vi "thrower Check for New Command.vi"(8 "Current Command":T6, 10 "Wait time (ms)":dbl, 11 "Finished?":bool) -> (0 "Completion":T4, 1 "Subsystem Name":string, 2 "Current Command":T1, 3 "Initial Trace String":string, 4 "NextCommand":T6)   [LabVIEW 2020]
doc: "This VI is called for each controller loop iteration. It checks for new commands, updates timing data, and upon completion, notifies any waiting commands."
uses:
  thrower Setpoints.ctl
  thrower Operations.ctl
  <vilib>/Rock Robotics/WPI/Framework/Command Status Info.ctl
  <vilib>/Rock Robotics/WPI/Framework/Completion Status.ctl
  <vilib>/Rock Robotics/WPI/Framework/Completion Notifier.ctl
  thrower Published Globals.vi
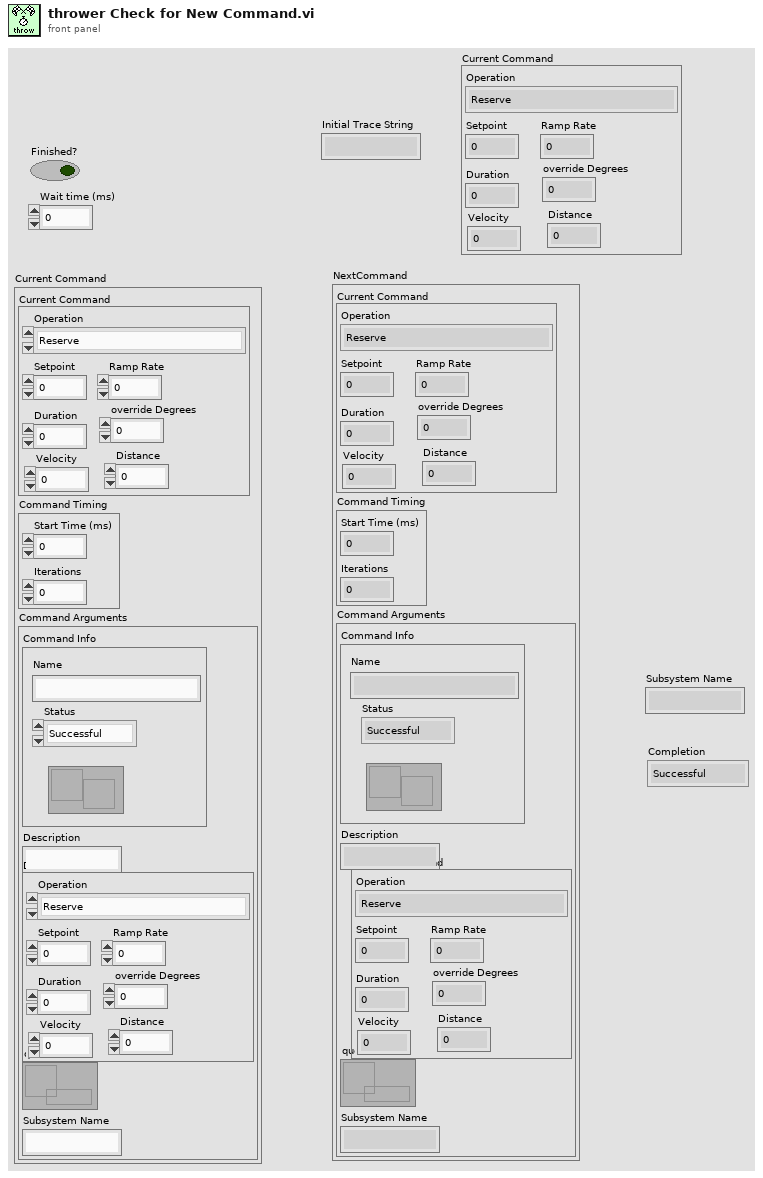
[diagram p1: front panel]
types:
  T1 = typedef "thrower Setpoints.ctl" = cluster{"Operation":T2, "Setpoint":dbl, "Duration":dbl, "Ramp Rate":dbl, "override Degrees":dbl, "Velocity":dbl, "Distance":dbl}
  T2 = typedef "thrower Operations.ctl" = enum16{"Reserve", "Read Current", "Immediate", "feed ball", "rev up thrower", "aim servos", "resetServos", "fire ball"}
  T3 = typedef "Command Status Info.ctl" = cluster{"Name":string, "Status":T4, "notifier out":T5}
  T4 = typedef "Completion Status.ctl" = enum16{"Successful", "Aborted", "Incomplete"}
  T5 = typedef "Completion Notifier.ctl" = refnum<notifier>
  T6 = cluster{"Current Command":T1, "Command Timing":cluster{"Start Time (ms)":u32, "Iterations":i32}, "Command Arguments":cluster{"Command Info":T3, "Description":string, "Default Command":T1, "queue out":refnum<queue>, "Subsystem Name":string}}
  T7 = cluster{"Command Info":T3, "Description":string, "Default Command":T1, "queue out":refnum<queue>, "Subsystem Name":string}
  T8 = cluster{"Default Command":T1, "Command Info":T3, "Description":string}
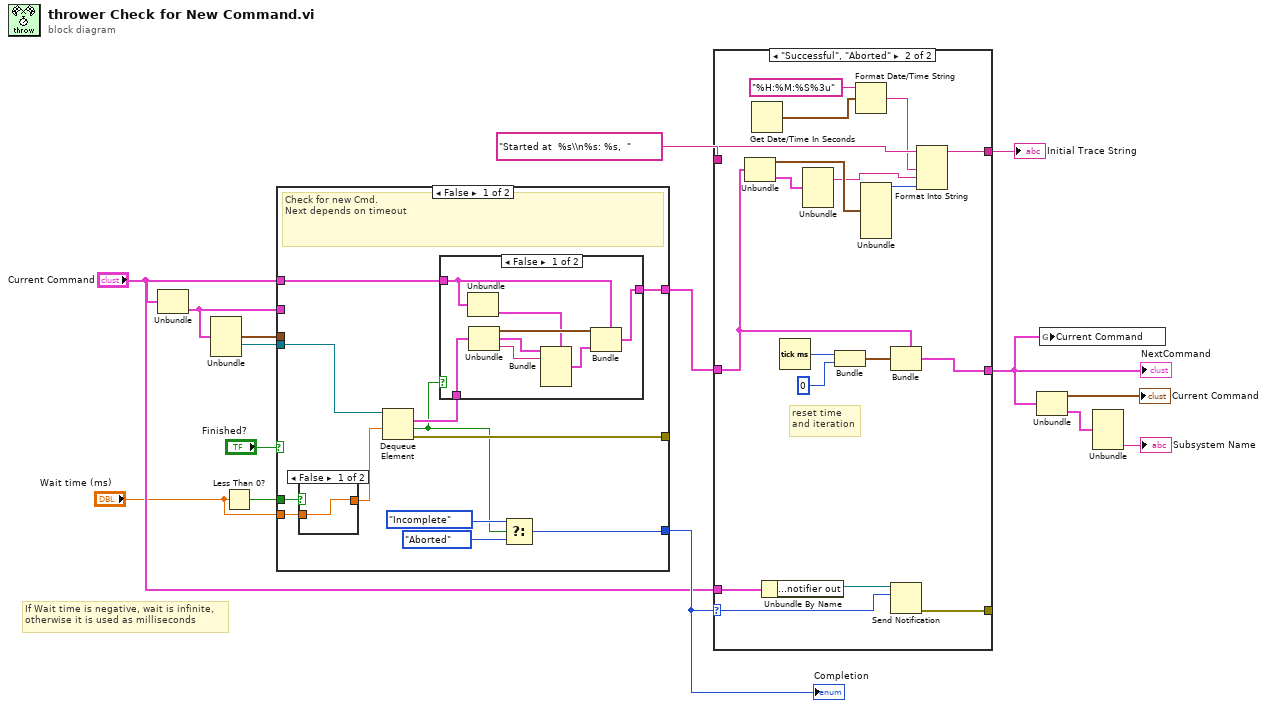
[diagram p0: block diagram]
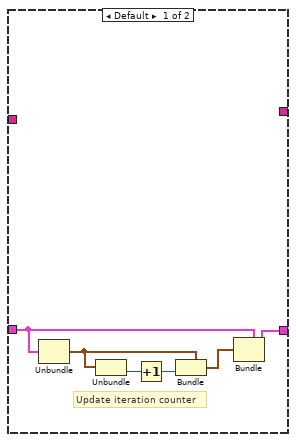
[diagram p2: hidden frame]
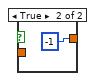
[diagram p4: hidden frame]
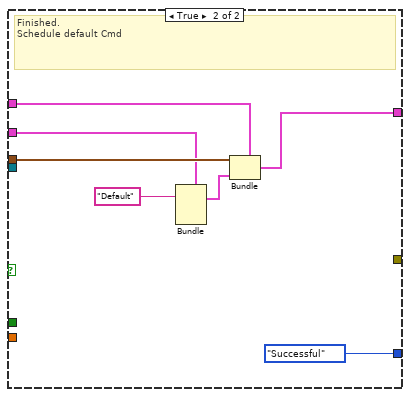
[diagram p5: hidden frame]
diagram:
  # "If Wait time is negative, wait is infinite,\notherwise it is used as milliseconds"
  n1 = Unbundle("Current Command") -> ("Command Arguments"=w4:T7)  [unwired: 2 out]
  n2 = Unbundle(w4) -> ("Default Command"=w7:T1, "queue out"=w8:refnum<queue>)  [unwired: 3 out]
  n3 = Less Than 0?(x="Wait time (ms)") -> (x < 0?=w2:bool)
  n4 = case shown="False" "Finished?" {
    tunnel: [w22 w44] -> w11
    tunnel: w2 -> [w24 _]
    tunnel: [w27 Completion_Status."Successful"] -> w15
    tunnel: [w19 _] -> _
    tunnel: w8 -> [w21 _]
    tunnel: "Current Command" -> [w23 w43]
    tunnel: w7 -> [_ w42]
    tunnel: w4 -> [_ w40]
    tunnel: "Wait time (ms)" -> [w16 _]
    frame False {
      # "Check for new Cmd.\nNext depends on timeout"
      n5 = case shown="False" w24 {
        tunnel: [w37 -1] -> w20
        tunnel: w16 -> [w37 _]
        frame False {
        }
        frame True {
        }
      }
      n6 = Dequeue Element(queue=w21, timeout in ms (-1)=w20) -> (element=w18:T8, timed out?=w17:bool, error out=w19:errorcluster)  [unwired: 1 in, 1 out]
      n7 = case shown="False" w17 {
        tunnel: w18 -> [w35 _]
        tunnel: w23 -> [w32 w36]
        tunnel: [w28 w36] -> w22
        frame False {
          n8 = Unbundle(w32) -> ("Command Arguments"=w31:T7)  [unwired: 2 out]
          n9 = Unbundle(w35) -> ("Default Command"=w34:T1, "Command Info"=w29:T3, "Description"=w30:string)
          n10 = Bundle(cluster=w31, "Command Info"=w29, "Description"=w30) -> (w33:T7)  [unwired: 3 in]
          n11 = Bundle(cluster=w32, "Current Command"=w34, "Command Arguments"=w33) -> (w28:T6)  [unwired: 1 in]
        }
        frame True {
        }
      }
      n12 = Select(t=Completion_Status."Incomplete", s=w17, f=Completion_Status."Aborted") -> (s? t:f=w27:T4)
    }
    frame True {
      # "Finished.\nSchedule default Cmd"
      n13 = Bundle(cluster=w40, "Description"="Default") -> (w41:T7)  [unwired: 4 in]
      n14 = Bundle(cluster=w43, "Current Command"=w42, "Command Arguments"=w41) -> (w44:T6)  [unwired: 1 in]
    }
  }
  "Completion" <- w15
  n15 = case shown="\"Successful\", \"Aborted\"" w15 {
    selector: w15 -> [_ w69]
    tunnel: "Current Command" -> [_ w66]
    tunnel: "Started at  %s\\n%s: %s,  " ("format string") -> [_ w65]
    tunnel: [_ w64] -> w13
    tunnel: w11 -> [w48 w53]
    tunnel: [w49 w60] -> w3
    tunnel: [_ w57] -> _
    frame Default {
      # "Update iteration counter"
      n16 = Unbundle(w48) -> ("Command Timing"=w47:cluster{"Start Time (ms)":u32, "Iterations":i32})  [unwired: 2 out]
      n17 = Unbundle(w47) -> ("Iterations"=w50:i32)  [unwired: 1 out]
      n18 = Increment(x=w50) -> (x+1=w51:i32)
      n19 = Bundle(cluster=w47, "Iterations"=w51) -> (w46:cluster{"Start Time (ms)":u32, "Iterations":i32})  [unwired: 1 in]
      n20 = Bundle(cluster=w48, "Command Timing"=w46) -> (w49:T6)  [unwired: 2 in]
    }
    frame "Successful", "Aborted" {
      # "reset time\nand iteration"
      n21 = Unbundle(w53) -> ("Current Command"=w63:T1, "Command Arguments"=w58:T7)  [unwired: 1 out]
      n22 = Get Date/Time In Seconds() -> (seconds since 1Jan1904=w56:timestamp)
      n23 = Unbundle By Name(w66) -> ("Command Arguments.Command Info.notifier out"=w68:T5)
      n24 = Tick Count (ms)() -> (millisecond timer value=w62:u32)
      n25 = Unbundle(w58) -> ("Description"=w55:string)  [unwired: 4 out]
      n26 = Bundle("millisecond timer value"=w62, 0) -> (w59:cluster{"millisecond timer value":u32, i32})  [unwired: 1 in]
      n27 = Format Date/Time String(time format string (%c)="%H:%M:%S%3u", seconds (now)=w56) -> (date/time string=w54:string)  [unwired: 1 in]
      n28 = Unbundle(w63) -> ("Operation"=w67:T2)  [unwired: 6 out]
      n29 = Bundle(cluster=w53, "Command Timing"=w59) -> (w60:T6)  [unwired: 2 in]
      n30 = Send Notification(notification=w69, notifier=w68) -> (error out=w57:errorcluster)  [unwired: 1 in, 1 out]
      n31 = Format Into String(format string=w65, w54, w55, w67) -> (resulting string=w64:string)  [unwired: 2 in, 1 out]
    }
  }
  "NextCommand" <- w3
  "Initial Trace String" <- w13
  n32 = Unbundle(w3) -> ("Current Command"=→"Current Command":T1, "Command Arguments"=w6:T7)  [unwired: 1 out]
  n33 = global write "thrower Published Globals.vi" "Current Command"(w3) -> ()
  n34 = Unbundle(w6) -> ("Subsystem Name"=→"Subsystem Name":string)  [unwired: 4 out]
